vi "VMS_3_Slave.vi"   [LabVIEW 2018]
uses:
  Common_FPGA_Timestamp/FPGATimestamp.lvlib
  Common_FPGA_Timestamp/DataTypes/TimestampSettings.ctl
  <vilib>/rvi/DataTransferAndStorage/Container/XNode/niFpgaContainer.xnode
  <vilib>/eio/EIONode/EIONode.xnode
  <vilib>/rvi/eio/common/nirviEmuTemplateMethod_errors.vi
  <vilib>/rvi/FIFO/Fifo_Resource/nirvififoEmulationRead.vi
  <vilib>/rvi/DataTransferAndStorage/Register/Emulation/niFpgaRegisterEmulation.vi
types:
  T1 = typedef "FPGATimestamp.lvlib/TimestampSettings.ctl" = cluster{"TimeSource":refnum<k21>, "TimeRegister":refnum<k21>, "IterationsPerMicrosecond":i16, "UpdateFIFO":refnum<k21>, "HealthAndStatusFIFO":refnum<k21>, "HealthAndStatusAddress":i16, "IterationsPerHealthAndStatusUpdate":i16}
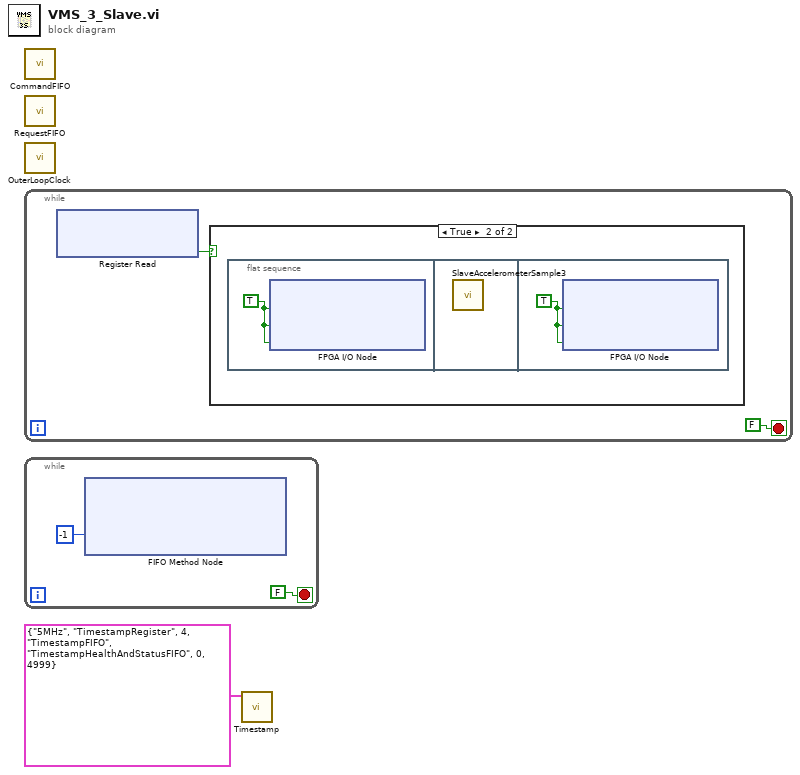
[diagram p0: block diagram]
diagram:
  n1 = call "CommandFIFO.vi"() -> ()  [unwired: 12 in]
  n2 = call "RequestFIFO.vi"() -> ()  [unwired: 12 in]
  n3 = call "OuterLoopClock.vi"() -> ()  [unwired: 12 in]
  n4 = while {
    stop <- FALSE stop-if-true
    n5 = xnode ("Register Read")() -> ("Data"=w2:bool)  [unwired: 1 in, 1 out]
    n6 = case shown="True" w2 {
      frame False {
      }
      frame True {
        n7 = flat-sequence {
          frame #0 {
            w4 = TRUE ("Accelerometer5/Start")
            n8 = xnode "FPGA I/O Node"("Accelerometer1/Start"=w4, "Accelerometer2/Start"=w4, "Accelerometer3/Start"=w4) -> ()  [unwired: 3 in, 3 out]
          }
          frame #1 {
            n9 = call "SlaveAccelerometerSample3.vi"() -> ()  [unwired: 12 in]
          }
          frame #2 {
            w5 = TRUE ("Accelerometer5/Start")
            n10 = xnode "FPGA I/O Node"("Accelerometer1/Stop"=w5, "Accelerometer2/Stop"=w5, "Accelerometer3/Stop"=w5) -> ()  [unwired: 3 in, 3 out]
          }
        }
      }
    }
  }
  n11 = while {
    stop <- FALSE stop-if-true
    n12 = xnode ("FIFO Method Node")("Timeout"=-1) -> ()  [unwired: 1 in, 3 out]
  }
  n13 = call "Timestamp.vi"("TimestampSettings"=T1 {"TimeSource"="5MHz", "TimeRegister"="TimestampRegister", "IterationsPerMicrosecond"=4, "UpdateFIFO"="TimestampFIFO", "HealthAndStatusFIFO"="TimestampHealthAndStatusFIFO", "HealthAndStatusAddress"=0, "IterationsPerHealthAndStatusUpdate"=4999}) -> ()  [unwired: 11 in]
